vi "Binary Data to Waveforms.vi"(0 "Binary Data":u8[](array[numeric])) -> (1 "Waveforms":T2, 2 "Meta":T1={"# Pages"=0, "ODR"=0, "xlRange"=0, "gyroRange"=0, "id"=0, "Samplig Freq [Hz]"=9.980607627666451, "xlRange in g"=0.0, "gyroRange in dps"=0.0} {"id" format="%02d"; "xlRange" format="%02x"; "ODR" format="%02x"})   [LabVIEW 2017]
uses:
  Controls/gyro_control_measurement_settings.ctl
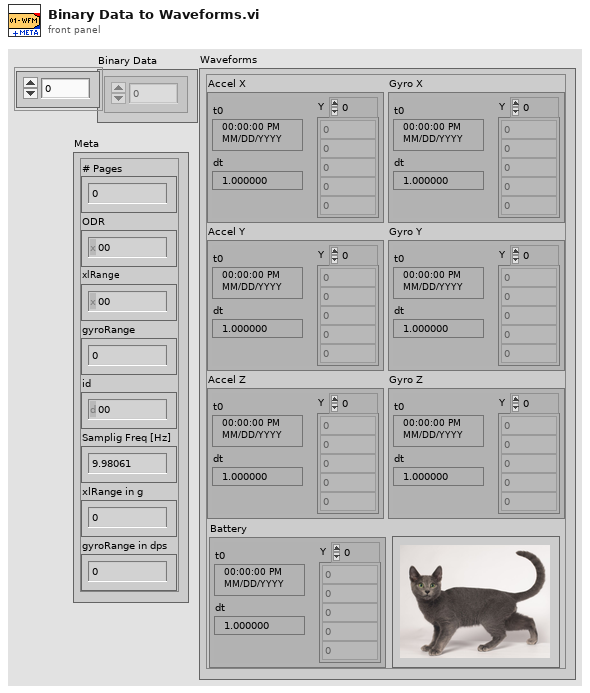
[diagram p1: front panel]
types:
  T1 = typedef "gyro_control_measurement_settings.ctl" = cluster{"# Pages":i32, "ODR":u8, "xlRange":u8, "gyroRange":u8, "id":u8, "Samplig Freq [Hz]":dbl, "xlRange in g":dbl, "gyroRange in dps":dbl}
  T2 = cluster{"Accel X":waveform(dbl), "Accel Y":waveform(dbl), "Accel Z":waveform(dbl), "Gyro X":waveform(dbl), "Gyro Y":waveform(dbl), "Gyro Z":waveform(dbl), "Battery":waveform(dbl)}
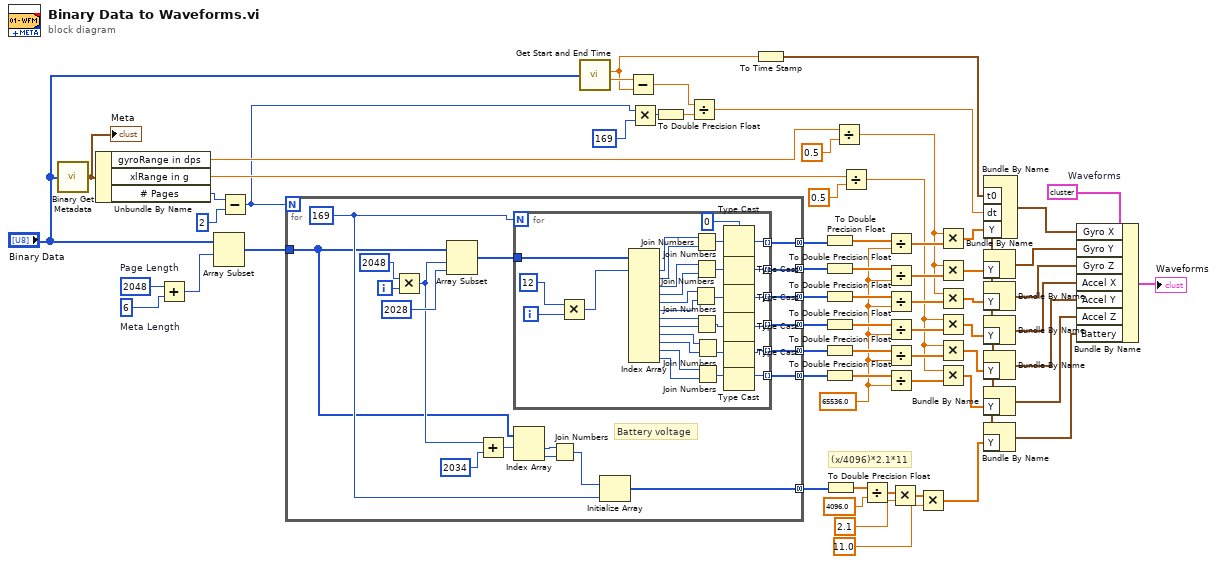
[diagram p0: block diagram]
diagram:
  w30 = T2 {"Accel X"={"t0"=timestamp(0 s since 1904-01-01), "dt"=1.0, "Y"=[]}, "Accel Y"={"t0"=timestamp(0 s since 1904-01-01), "dt"=1.0, "Y"=[]}, "Accel Z"={"t0"=timestamp(0 s since 1904-01-01), "dt"=1.0, "Y"=[]}, "Gyro X"={"t0"=timestamp(0 s since 1904-01-01), "dt"=1.0, "Y"=[]}, "Gyro Y"={"t0"=timestamp(0 s since 1904-01-01), "dt"=1.0, "Y"=[]}, "Gyro Z"={"t0"=timestamp(0 s since 1904-01-01), "dt"=1.0, "Y"=[]}, "Battery"={"t0"=timestamp(0 s since 1904-01-01), "dt"=1.0, "Y"=[]}}  # Waveforms
  w49 = 65536.0 ("y")
  w63 = 2048  # Page Length
  w62 = 6  # Meta Length
  # "(x/4096)*2.1*11"
  n1 = call "Binary Get Metadata.vi"("Binary Data"="Binary Data") -> ("Meta"=w1:T1)  [unwired: 4 in]
  "Meta" <- w1
  n2 = Unbundle By Name(w1) -> ("gyroRange in dps"=w19:dbl, "xlRange in g"=w15:dbl, "# Pages"=w22:i32)
  n3 = Add(x=w63, y=w62) -> (x+y=w64:i32)
  n4 = Array Subset(array="Binary Data", index=w64) -> (w65:u8[])  [unwired: 1 in]
  n5 = Subtract(x=w22, y=2) -> (x-y=w3:i32)
  n6 = for {
    N: w3 -> [_]
    tunnel: w65 -> [w71]
    tunnel: [w81] -> w61 mode=concatenating
    tunnel: [w80] -> w60 mode=concatenating
    tunnel: [w79] -> w59 mode=concatenating
    tunnel: [w78] -> w58 mode=concatenating
    tunnel: [w77] -> w57 mode=concatenating
    tunnel: [w76] -> w56 mode=concatenating
    tunnel: [w68] -> w12 mode=concatenating
    i -> [w84]
    w74 = 169
    # "Battery voltage"
    n7 = Multiply(x=2048, y=w84) -> (x*y=w72:i32)
    n8 = Array Subset(array=w71, index=w72, length=2028) -> (w73:u8[])
    n9 = Add(x=w72, y=2034 ("length")) -> (x+y=w66:i32)
    n10 = for {
      N: w74 -> [_]
      tunnel: w73 -> [w111]
      tunnel: [w90] -> w81 mode=indexing
      tunnel: [w96] -> w80 mode=indexing
      tunnel: [w95] -> w79 mode=indexing
      tunnel: [w94] -> w78 mode=indexing
      tunnel: [w93] -> w77 mode=indexing
      tunnel: [w92] -> w76 mode=indexing
      i -> [w113]
      w91 = i16 0
      n11 = Multiply(x=12, y=w113) -> (x*y=w110:i32)
      n12 = Index Array(array=w111, index #1=w110) -> (element #1=w109:u8, element #2=w108:u8, element #3=w107:u8, element #4=w106:u8, element #5=w105:u8, element #6=w104:u8, element #7=w103:u8, element #8=w102:u8, element #9=w101:u8, element #10=w100:u8, element #11=w99:u8, element #12=w98:u8)  [unwired: 11 in]
      n13 = Join Numbers(hi=w105, lo=w104) -> ((hi.lo)=w88:u16)
      n14 = Join Numbers(hi=w109, lo=w108) -> ((hi.lo)=w97:u16)
      n15 = Join Numbers(hi=w107, lo=w106) -> ((hi.lo)=w89:u16)
      n16 = Join Numbers(hi=w103, lo=w102) -> ((hi.lo)=w87:u16)
      n17 = Join Numbers(hi=w101, lo=w100) -> ((hi.lo)=w86:u16)
      n18 = Join Numbers(hi=w99, lo=w98) -> ((hi.lo)=w85:u16)
      n19 = Type Cast(type=w91, x=w97) -> (*(type *) &x=w90:i16)
      n20 = Type Cast(type=w91, x=w89) -> (*(type *) &x=w96:i16)
      n21 = Type Cast(type=w91, x=w88) -> (*(type *) &x=w95:i16)
      n22 = Type Cast(type=w91, x=w87) -> (*(type *) &x=w94:i16)
      n23 = Type Cast(type=w91, x=w86) -> (*(type *) &x=w93:i16)
      n24 = Type Cast(type=w91, x=w85) -> (*(type *) &x=w92:i16)
    }
    n25 = Index Array(array=w71, index #1=w66) -> (element #1=w70:u8, element #2=w69:u8)  [unwired: 1 in]
    n26 = Join Numbers(hi=w70, lo=w69) -> ((hi.lo)=w67:u16)
    n27 = Initialize Array(w67, w74) -> (w68:u16[])
  }
  n28 = call "Get Start and End Time.vi"("Binary Data"="Binary Data") -> ("Start Time"=w20:dbl, "End Time"=w21:dbl)  [unwired: 8 in]
  n29 = Subtract(x=w21, y=w20) -> (x-y=w42:dbl)
  n30 = Multiply(x=w3, y=169) -> (x*y=w40:i32)
  n31 = To Double Precision Float(number=w40) -> (double precision float=w41:dbl)
  n32 = Divide(x=w42, y=w41) -> (x/y=w32:dbl)
  n33 = To Time Stamp(1:w20) -> (0:w31:timestamp)
  n34 = To Double Precision Float(number=w61) -> (double precision float=w55:dbl[])
  n35 = To Double Precision Float(number=w60) -> (double precision float=w50:dbl[])
  n36 = To Double Precision Float(number=w59) -> (double precision float=w51:dbl[])
  n37 = To Double Precision Float(number=w58) -> (double precision float=w52:dbl[])
  n38 = To Double Precision Float(number=w57) -> (double precision float=w53:dbl[])
  n39 = To Double Precision Float(number=w56) -> (double precision float=w54:dbl[])
  n40 = To Double Precision Float(number=w12) -> (double precision float=w11:dbl[])
  n41 = Divide(x=w19, y=0.5) -> (x/y=w18:dbl)
  n42 = Divide(x=w15, y=0.5) -> (x/y=w14:dbl)
  n43 = Divide(x=w11, y=4096.0) -> (x/y=w9:dbl[])
  n44 = Divide(x=w55, y=w49) -> (x/y=w48:dbl[])
  n45 = Divide(x=w50, y=w49) -> (x/y=w47:dbl[])
  n46 = Divide(x=w51, y=w49) -> (x/y=w46:dbl[])
  n47 = Divide(x=w52, y=w49) -> (x/y=w45:dbl[])
  n48 = Divide(x=w53, y=w49) -> (x/y=w43:dbl[])
  n49 = Divide(x=w54, y=w49) -> (x/y=w44:dbl[])
  n50 = Multiply(x=w9, y=2.1) -> (x*y=w8:dbl[])
  n51 = Multiply(x=w8, y=11.0) -> (x*y=w5:dbl[])
  n52 = Multiply(x=w18, y=w48) -> (x*y=w33:dbl[])
  n53 = Multiply(x=w18, y=w47) -> (x*y=w34:dbl[])
  n54 = Multiply(x=w18, y=w46) -> (x*y=w35:dbl[])
  n55 = Multiply(x=w14, y=w45) -> (x*y=w36:dbl[])
  n56 = Multiply(x=w14, y=w43) -> (x*y=w37:dbl[])
  n57 = Multiply(x=w14, y=w44) -> (x*y=w38:dbl[])
  n58 = Bundle By Name("t0"=w31, "dt"=w32, "Y"=w33) -> (w2:waveform(dbl))  [unwired: 1 in]
  n59 = Bundle By Name(cluster=w2, "Y"=w34) -> (w25:waveform(dbl))
  n60 = Bundle By Name(cluster=w2, "Y"=w35) -> (w26:waveform(dbl))
  n61 = Bundle By Name(cluster=w2, "Y"=w36) -> (w27:waveform(dbl))
  n62 = Bundle By Name(cluster=w2, "Y"=w37) -> (w28:waveform(dbl))
  n63 = Bundle By Name(cluster=w2, "Y"=w38) -> (w29:waveform(dbl))
  n64 = Bundle By Name(cluster=w2, "Y"=w5) -> (w4:waveform(dbl))
  n65 = Bundle By Name(cluster=w30, "Gyro X"=w2, "Gyro Y"=w25, "Gyro Z"=w26, "Accel X"=w27, "Accel Y"=w28, "Accel Z"=w29, "Battery"=w4) -> (→"Waveforms":T2)
